vi "ftngen2.vi"() -> ()   [LabVIEW 2019]
uses:
  <vilib>/measure/NI_MABase.lvlib
panel:
  out "Waveform Graph":waveform(dbl)(graph)
  in  "?":string
  out "?":string
  in  "DC/AC":enum16{"AC", "DC"}(ring)
  in  "DC Offset":dbl(knob) scale=0.0..10.0
  in  "x100":bool
  in  "x1K":bool
  out "?":dbl
  in  "Frequency":dbl(knob) scale=0.0..10.0
  in  "Amplitude":dbl(knob) scale=0.0..10.0
  in  "전원":bool
  out "?":bool
  # "[Hz]"
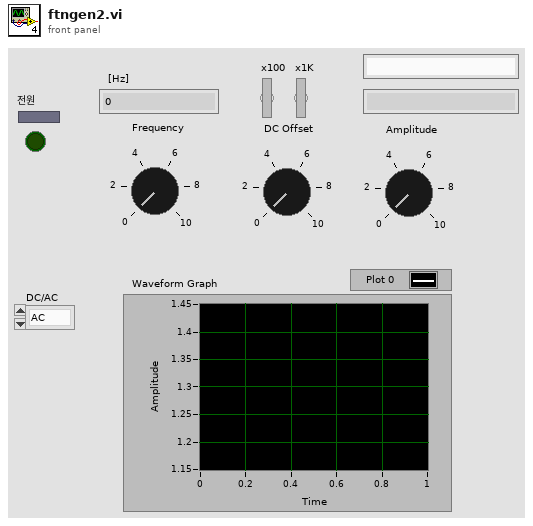
[diagram p1: front panel]
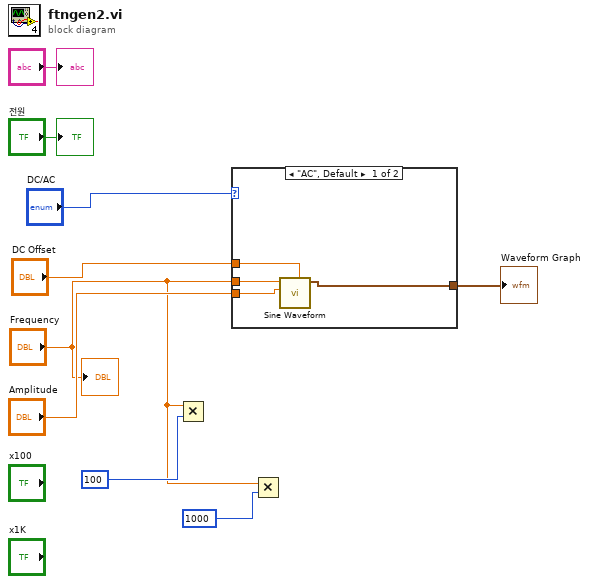
[diagram p0: block diagram]
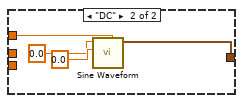
[diagram p2: hidden frame]
diagram:
  n1 = Multiply(x="Frequency", y=100) -> ()  [unwired: 1 out]
  n2 = case shown="\"AC\", Default" "DC/AC" {
    tunnel: "DC Offset" -> [w13 w17]
    tunnel: "Amplitude" -> [w12 _]
    tunnel: "Frequency" -> [w11 _]
    tunnel: [w10 w16] -> w4
    frame "AC", Default {
      n3 = call <vilib>:"Sine Waveform.vi"("offset"=w13, "amplitude"=w12, "frequency"=w11) -> ("signal out"=w10:waveform(dbl))  [unwired: 7 in, 1 out]
    }
    frame "DC" {
      n4 = call <vilib>:"Sine Waveform.vi"("offset"=w17, "amplitude"=0.0, "frequency"=0.0) -> ("signal out"=w16:waveform(dbl))  [unwired: 7 in, 1 out]
    }
  }
  "Waveform Graph" <- w4
  n5 = Multiply(x="Frequency", y=1000) -> ()  [unwired: 1 out]
  "?" <- "전원"
  "?" <- "?"
  "?" <- "Frequency"
